vi "RetrieveDefaultPathData.vi"(8 "error in (no error)":errorcluster, 10 "Path":path, 11 "Setting Database In":refnum<class "Setting Database.lvclass">) -> (0 "error out":errorcluster, 2 "Path Settings":refnum<class "Path Settings.lvclass">, 3 "Setting Database Out":refnum<class "Setting Database.lvclass">)   [LabVIEW 2019, in "Setting Database.lvclass"]
uses:
  Setting Database.lvclass
  Path Settings/Path Settings.lvclass
  Setting Database.lvclass/Setting Database.ctl
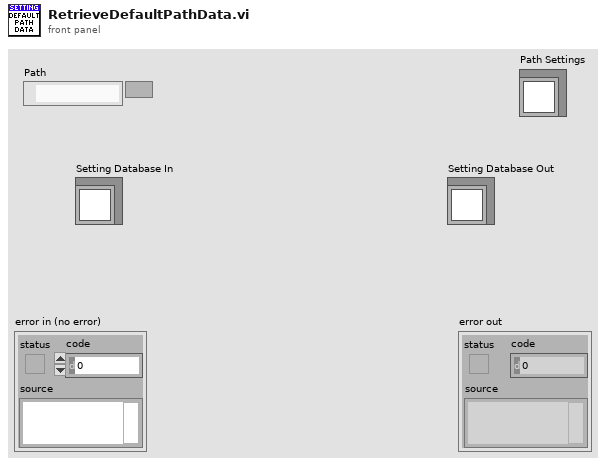
[diagram p1: front panel]
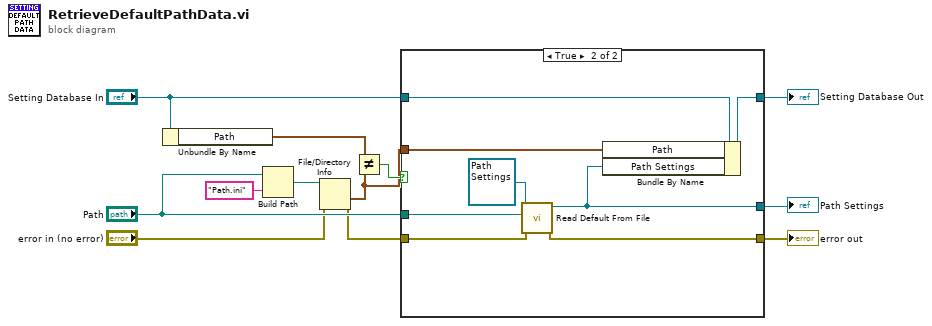
[diagram p0: block diagram]
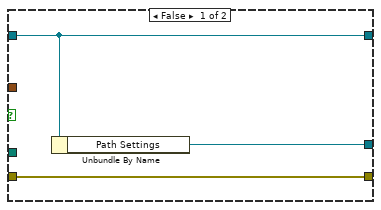
[diagram p2: hidden frame]
diagram:
  n1 = Unbundle By Name("Setting Database In") -> ("Path"=w2:timestamp)
  n2 = Build Path(base path="Path", name or relative path="Path.ini") -> (appended path=w9:path)
  n3 = File/Directory Info(path=w9, error in="error in (no error)") -> (last mod=w1:timestamp, error out=w3:errorcluster)  [unwired: 5 out]
  n4 = Not Equal?(x=w2, y=w1) -> (x != y?=w7:bool)
  n5 = case shown="True" w7 {
    tunnel: [w15 w17] -> w11
    tunnel: "Path" -> [_ w23]
    tunnel: "Setting Database In" -> [w14 w21]
    tunnel: [w14 w22] -> w12
    tunnel: w3 -> [w13 w18]
    tunnel: [w13 w19] -> w10
    tunnel: w1 -> [_ w16]
    frame False {
      n6 = Unbundle By Name(w14) -> ("Path Settings"=w15:refnum<class "Path Settings.lvclass">)
    }
    frame True {
      n7 = call-dynamic "Read Default From File.vi"("error in (no error)"=w18, "Path"=w23, "Path Settings in"=refnum<class "Path Settings.lvclass"> refnum) -> ("error out"=w19:errorcluster, "Path Settings out"=w17:refnum<class "Path Settings.lvclass">)  [unwired: 7 in]
      n8 = Bundle By Name(cluster=w21, "Path"=w16, "Path Settings"=w17) -> (w22:refnum<class "Setting Database.lvclass">)
    }
  }
  "error out" <- w10
  "Path Settings" <- w11
  "Setting Database Out" <- w12
